vi "Keithley Control Panel.vi"() -> ()   [LabVIEW 2017]
uses:
  Global/GPIB Numbers.vi
panel:
  in  "Reset Values":bool
  out "Numeric":i32
  in  "stop":bool
  in  "reference value (volts)":dbl min=-1100.0 max=1100.0 format="%^.2e"
  in  "reference (off:0)":u16(ring) items=["off", "set reference value"]
  in  "noise tolerance (%)":dbl=1.0 min=0.0 max=100.0 step=1.0 format="%^.2e"
  in  "advanced filter (off:0)":u16(ring) items=["off", "enabled"]
  in  "digital filter (off:0)":u16(ring) items=["off", "auto filter", "auto filter once", "moving filter", "repeating filter"]
  in  "dig. filter count":dbl=10.0 min=1.0 max=100.0 step=1.0 format="%^.2e"
  in  "range (auto:0)":u16(ring) items=["autorange", "autorange once", "set min range", "set max range", "set range value"]
  in  "range value (volts)":dbl=1000.0 min=0.2 max=1000.0 format="%^.2e"
  in  "resolution (4.5 digits:3)":u16(ring)=3 items=["auto resolution", "auto resolution once", "3.5 digits", "4.5 digits", "5.5 digits", "6.5 digits", "7.5 digits", "8.5 digits"]
  in  "integ. value":dbl=0.01667 format="%^.2e"
  in  "integration time (0:auto)":u16(ring) items=["automatic", "automatic once", "set to minimum", "set to maximum", "set aperature value", "set NPLC value"]
  out "error out":T1
  out "Reading Result":string
  in  "error in":T1
  in  "function (Vdc:1)":u16(ring)=1 items=["ac voltage", "dc voltage", "2-wire resistance", "4-wire resistance", "ac current", "dc current", "frequency", "temperature"]
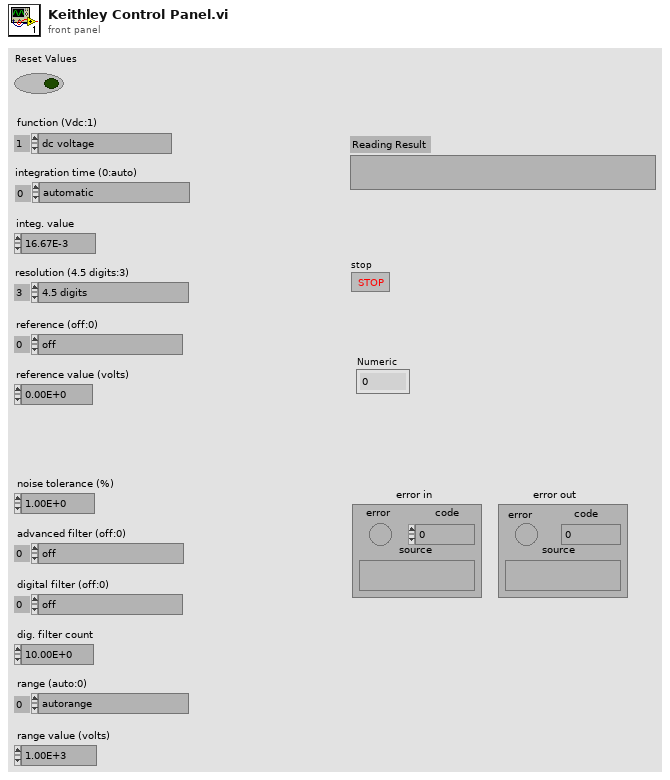
[diagram p1: front panel]
types:
  T1 = cluster{"error":bool, "code":i32, "source":string}
  T2 = typedef "GPIB Type Def.ctl" = cluster{"Name":string, "bus":dbl, "GPIB":dbl, "GPIB as string":string, "byte":i32, "VISA Resource Name":refnum<visa-resource-name>}
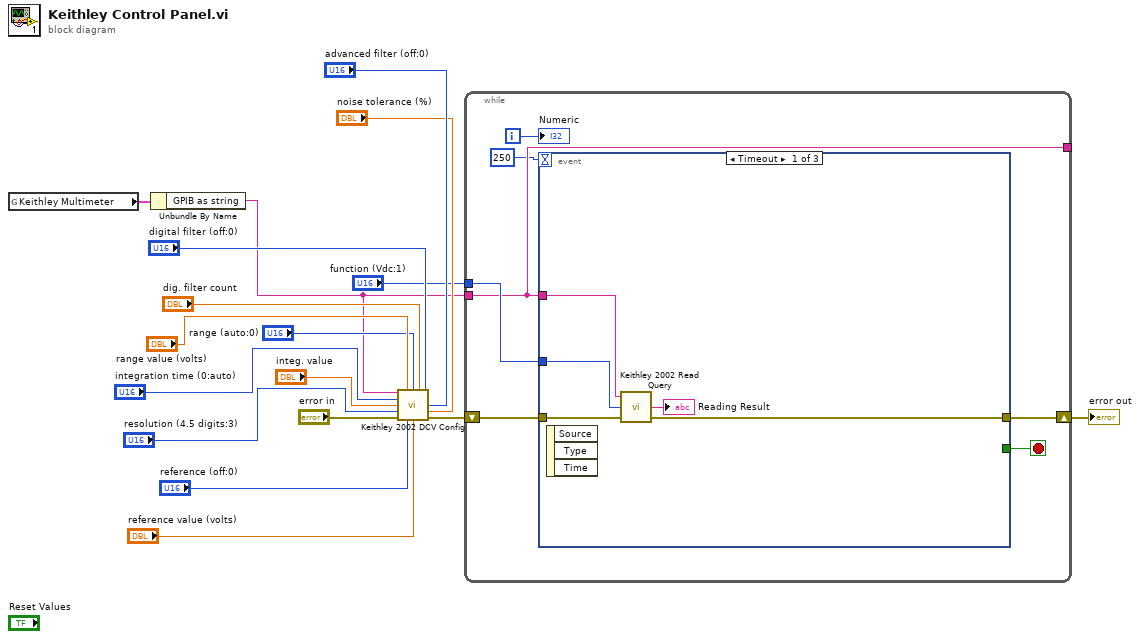
[diagram p0: block diagram]
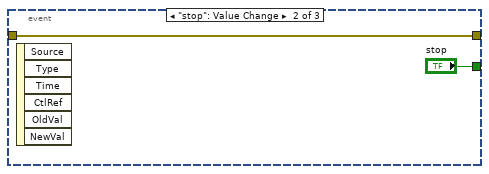
[diagram p2: hidden frame]
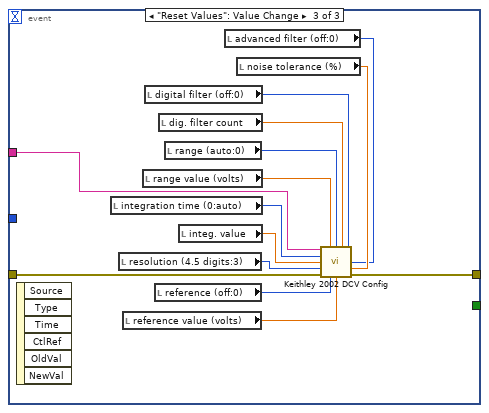
[diagram p3: hidden frame]
diagram:
  n1 = global read "GPIB Numbers.vi" "Keithley Multimeter"() -> (w5:T2)
  n2 = Unbundle By Name(w5) -> ("GPIB as string"=w1:string)
  n3 = call "Keithley 2002 DCV Config.vi"("GPIB address"=w1, "range value (volts)"="range value (volts)", "range (auto:0)"="range (auto:0)", "dig. filter count"="dig. filter count", "digital filter (off:0)"="digital filter (off:0)", "integration time (0:auto)"="integration time (0:auto)", "integ. value"="integ. value", "advanced filter (off:0)"="advanced filter (off:0)", "resolution (4.5 digits:3)"="resolution (4.5 digits:3)", "noise tolerance (%)"="noise tolerance (%)", "error in"="error in", "reference (off:0)"="reference (off:0)", "reference value (volts)"="reference value (volts)") -> ("error out"=w4:T1)  [unwired: 2 in]
  n4 = while {
    shift-right: [w19] -> w3
    shift-left: w4 -> [w20]
    tunnel: "function (Vdc:1)" -> [w22]
    tunnel: w1 -> [w21]
    tunnel: [w21] -> _
    i -> [w23]
    stop <- w24 stop-if-true
    n5 = event shown="[0] Timeout" {
      selector: _ -> [_ _ _]
      dyn-events: _ -> [_ _ _]
      timeout: 250 -> [_ _ _]
      tunnel: w20 -> [w26 w30 w33]
      tunnel: [w25 w30 w32] -> w19
      tunnel: [_ "stop" _] -> w24
      tunnel: w22 -> [w28 _ _]
      tunnel: w21 -> [w29 _ w34]
      event Timeout {
        n6 = event-data() -> ()  [unwired: 1 in, 3 out]
        n7 = call "Keithley 2002 Read Query.vi"("error in"=w26, "function (Vdc:1)"=w28, "GPIB Address"=w29) -> ("error out"=w25:T1, "Reading Result"=→"Reading Result":string)  [unwired: 1 in]
      }
      event "stop": Value Change {
        n8 = event-data() -> ()  [unwired: 1 in, 6 out]
      }
      event "Reset Values": Value Change {
        n9 = event-data() -> ()  [unwired: 1 in, 6 out]
        n10 = local read "integration time (0:auto)"() -> (w40:u16)
        n11 = local read "resolution (4.5 digits:3)"() -> (w39:u16)
        n12 = local read "reference value (volts)"() -> (w37:dbl)
        n13 = local read "range value (volts)"() -> (w45:dbl)
        n14 = local read "digital filter (off:0)"() -> (w42:u16)
        n15 = local read "reference (off:0)"() -> (w38:u16)
        n16 = local read "dig. filter count"() -> (w43:dbl)
        n17 = local read "range (auto:0)"() -> (w44:u16)
        n18 = local read "integ. value"() -> (w41:dbl)
        n19 = local read "advanced filter (off:0)"() -> (w35:u16)
        n20 = local read "noise tolerance (%)"() -> (w36:dbl)
        n21 = call "Keithley 2002 DCV Config.vi"("GPIB address"=w34, "range value (volts)"=w45, "range (auto:0)"=w44, "dig. filter count"=w43, "digital filter (off:0)"=w42, "integration time (0:auto)"=w40, "integ. value"=w41, "advanced filter (off:0)"=w35, "resolution (4.5 digits:3)"=w39, "noise tolerance (%)"=w36, "error in"=w33, "reference (off:0)"=w38, "reference value (volts)"=w37) -> ("error out"=w32:T1)  [unwired: 2 in]
      }
    }
    "Numeric" <- w23
  }
  "error out" <- w3
